vi "Atividade 3.vi"() -> ()   [LabVIEW 2015]
panel:
  in  "Numeric":dbl
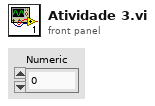
[diagram p1: front panel]
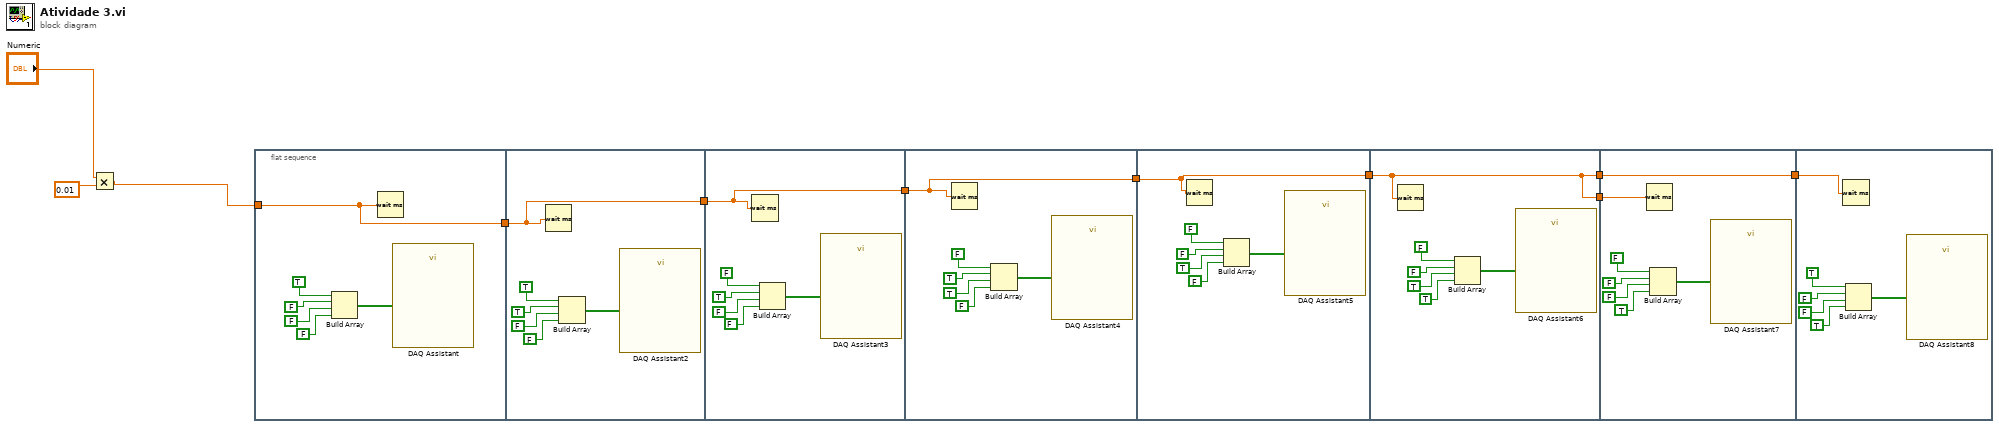
[diagram p0: block diagram]
diagram:
  n1 = Multiply(x="Numeric", y=0.01) -> (x*y=w3:dbl)
  n2 = flat-sequence {
    tunnel: w3 -> [w12]
    tunnel: [w12] -> w11
    tunnel: w11 -> [w18]
    tunnel: [w18] -> w10
    tunnel: w10 -> [w24]
    tunnel: [w24] -> w9
    tunnel: w9 -> [w30]
    tunnel: [w30] -> w8
    tunnel: w8 -> [w36]
    tunnel: [w36] -> w7
    tunnel: w7 -> [w42]
    tunnel: [w42] -> w6
    tunnel: [w42] -> w5
    tunnel: w6 -> [w49]
    tunnel: w5 -> [w48]
    tunnel: [w48] -> w4
    tunnel: w4 -> [w55]
    frame #0 {
      n3 = Build Array(TRUE, FALSE, FALSE, FALSE) -> (w13:bool[])
      n4 = Wait (ms)(milliseconds to wait=w12) -> ()  [unwired: 1 out]
      n5 = call "DAQ Assistant"("data"=w13) -> ()  [unwired: 17 in, 2 out]
    }
    frame #1 {
      n6 = Wait (ms)(milliseconds to wait=w18) -> ()  [unwired: 1 out]
      n7 = Build Array(TRUE, TRUE, FALSE, FALSE) -> (w19:bool[])
      n8 = call "DAQ Assistant2"("data"=w19) -> ()  [unwired: 17 in, 2 out]
    }
    frame #2 {
      n9 = Wait (ms)(milliseconds to wait=w24) -> ()  [unwired: 1 out]
      n10 = Build Array(FALSE, TRUE, FALSE, FALSE) -> (w25:bool[])
      n11 = call "DAQ Assistant3"("data"=w25) -> ()  [unwired: 17 in, 2 out]
    }
    frame #3 {
      n12 = Wait (ms)(milliseconds to wait=w30) -> ()  [unwired: 1 out]
      n13 = Build Array(FALSE, TRUE, TRUE, FALSE) -> (w31:bool[])
      n14 = call "DAQ Assistant4"("data"=w31) -> ()  [unwired: 17 in, 2 out]
    }
    frame #4 {
      n15 = Wait (ms)(milliseconds to wait=w36) -> ()  [unwired: 1 out]
      n16 = Build Array(FALSE, FALSE, TRUE, FALSE) -> (w37:bool[])
      n17 = call "DAQ Assistant5"("data"=w37) -> ()  [unwired: 17 in, 2 out]
    }
    frame #5 {
      n18 = Wait (ms)(milliseconds to wait=w42) -> ()  [unwired: 1 out]
      n19 = Build Array(FALSE, FALSE, TRUE, TRUE) -> (w43:bool[])
      n20 = call "DAQ Assistant6"("data"=w43) -> ()  [unwired: 17 in, 2 out]
    }
    frame #6 {
      n21 = Wait (ms)(milliseconds to wait=w49) -> ()  [unwired: 1 out]
      n22 = Build Array(FALSE, FALSE, FALSE, TRUE) -> (w50:bool[])
      n23 = call "DAQ Assistant7"("data"=w50) -> ()  [unwired: 17 in, 2 out]
    }
    frame #7 {
      n24 = Wait (ms)(milliseconds to wait=w55) -> ()  [unwired: 1 out]
      n25 = Build Array(TRUE, FALSE, FALSE, TRUE) -> (w56:bool[])
      n26 = call "DAQ Assistant8"("data"=w56) -> ()  [unwired: 17 in, 2 out]
    }
  }
